vi "RW_RobotCalsALB.vi"(7 "Action":enum16{"read", "write"}(ring), 10 "Settings":T1, 11 "File Path":path=path "c:/Robot.cfg") -> (0 "error out":errorcluster, 2 "Settings out":T1)   [LabVIEW 2017]
uses:
  CtrlRefs/SettingsALB.ctl
  <vilib>/Utility/config.llb/Read Key (Double).vi
  <vilib>/Utility/config.llb/Write Key (Double).vi
  <vilib>/Utility/config.llb/NI_LVConfig.lvlib
panel:
  in  "Tab Control":enum32{"Inputs", "Outputs"}(tab)
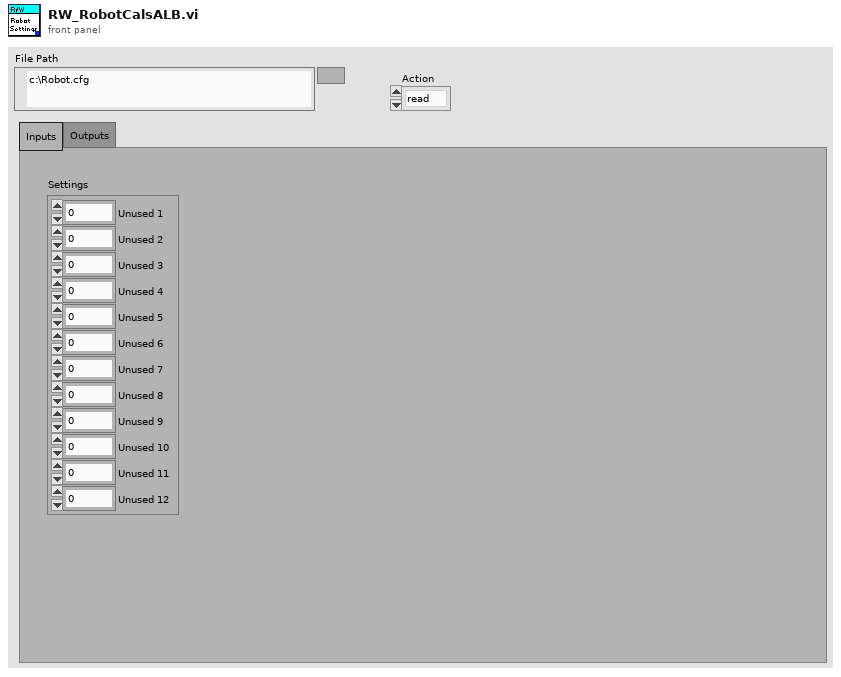
[diagram p1: front panel]
types:
  T1 = typedef "SettingsALB.ctl" = cluster{"Unused 1":dbl, "Unused 2":dbl, "Unused 3":dbl, "Unused 4":dbl, "Unused 5":dbl, "Unused 6":dbl, "Unused 7":dbl, "Unused 8":dbl, "Unused 9":dbl, "Unused 10":dbl, "Unused 11":dbl, "Unused 12":dbl}
  T2 = typedef "NI_LVConfig.lvlib/Config Data RefNum.ctl" = refnum<k1>
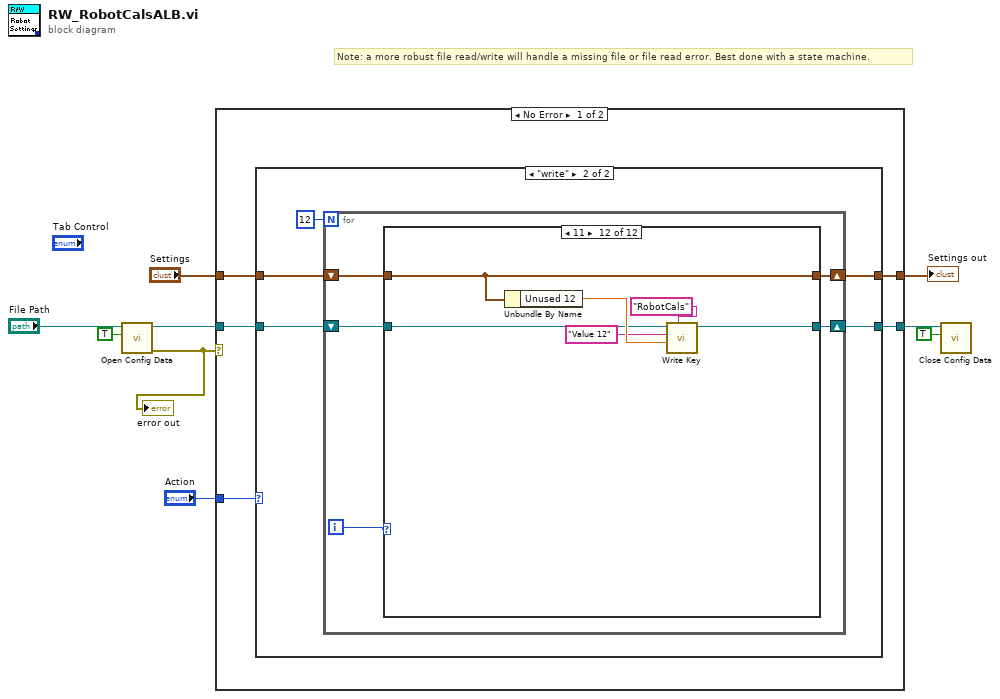
[diagram p0: block diagram]
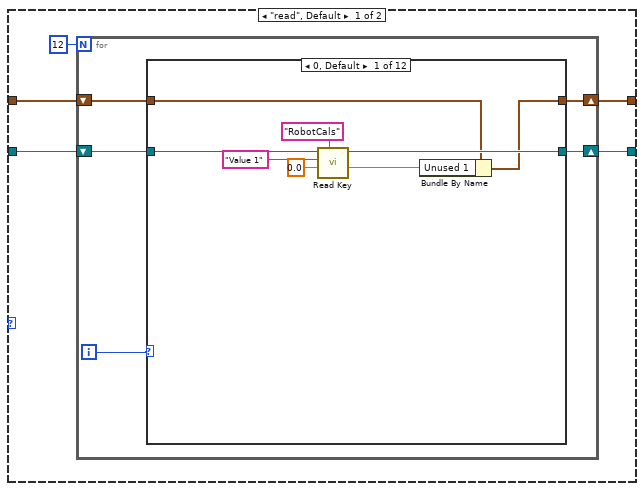
[diagram p2: hidden frame]
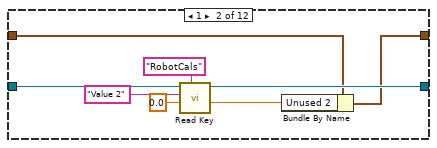
[diagram p3: hidden frame]
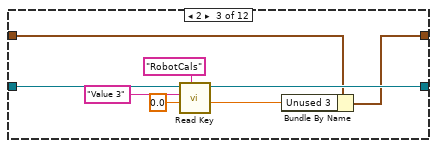
[diagram p4: hidden frame]
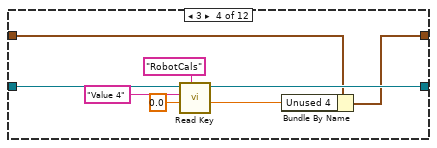
[diagram p5: hidden frame]
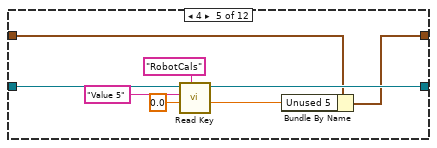
[diagram p6: hidden frame]
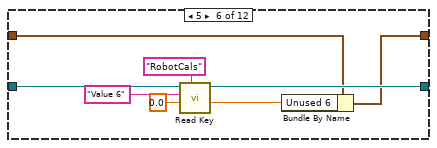
[diagram p7: hidden frame]
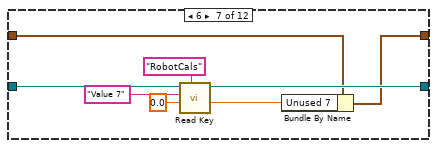
[diagram p8: hidden frame]
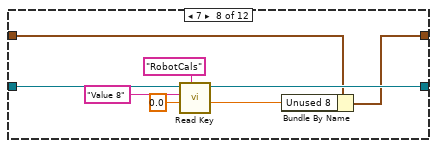
[diagram p9: hidden frame]
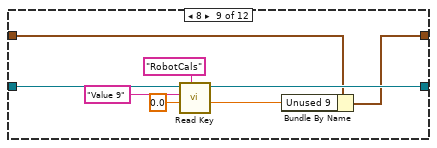
[diagram p10: hidden frame]
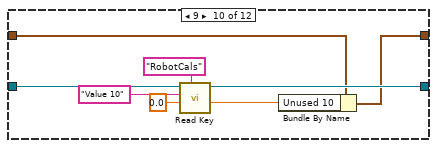
[diagram p11: hidden frame]
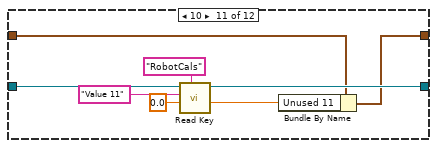
[diagram p12: hidden frame]
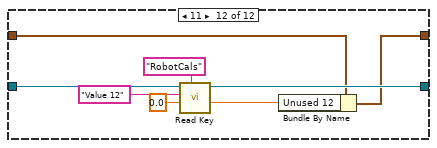
[diagram p13: hidden frame]
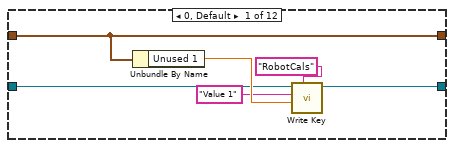
[diagram p14: hidden frame]
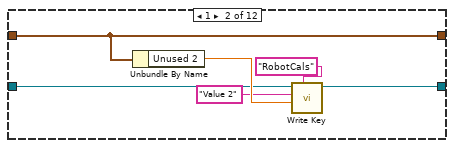
[diagram p15: hidden frame]
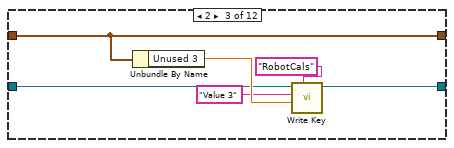
[diagram p16: hidden frame]
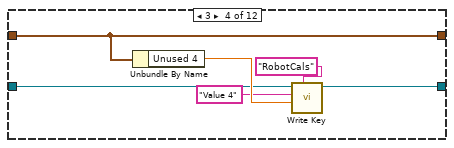
[diagram p17: hidden frame]
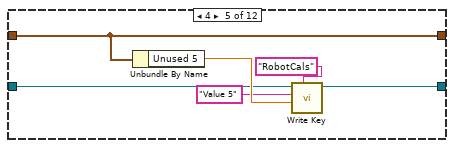
[diagram p18: hidden frame]
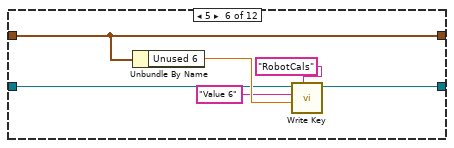
[diagram p19: hidden frame]
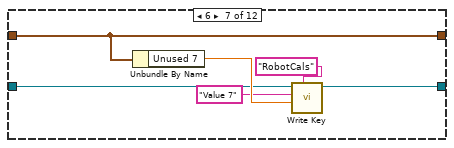
[diagram p20: hidden frame]
diagram:
  # "Note: a more robust file read/write will handle a missing file or file read error. Best done with a state machine."
  n1 = call <vilib>:"Open Config Data.vi"("create file if necessary (T)"=TRUE, "configuration file path"="File Path") -> ("error out"=w5:errorcluster, "refnum"=w7:T2)  [unwired: 7 in, 1 out]
  "error out" <- w5
  n2 = case shown="No Error" w5 {
    tunnel: "Action" -> [w14 _]
    tunnel: w7 -> [w13 w203]
    tunnel: "Settings" -> [w12 w204]
    tunnel: [w11 w204] -> w1
    tunnel: [w10 w203] -> w3
    frame No Error {
      n3 = case shown="\"write\"" w14 {
        tunnel: w13 -> [w19 w125]
        tunnel: w12 -> [w18 w124]
        tunnel: [w17 w123] -> w11
        tunnel: [w15 w121] -> w10
        frame "read", Default {
          n4 = for {
            N: 12 -> [_]
            shift-right: [w20] -> w17
            shift-left: w18 -> [w21]
            shift-right: [w22] -> w15
            shift-left: w19 -> [w23]
            i -> [w24]
            n5 = case shown="0, Default" w24 {
              tunnel: w23 -> [w28 w36 w44 w52 w60 w68 w76 w84 w92 w100 w108 w116]
              tunnel: [w27 w35 w43 w51 w59 w67 w75 w83 w91 w99 w107 w115] -> w22
              tunnel: w21 -> [w26 w34 w42 w50 w58 w66 w74 w82 w90 w98 w106 w114]
              tunnel: [w25 w33 w41 w49 w57 w65 w73 w81 w89 w97 w105 w113] -> w20
              frame 0, Default {
                n6 = call-poly <vilib>:"Read Key.vi"("section"="RobotCals", "default value"=0.0, "key"="Value 1" ("section"), "refnum"=w28) -> ("value"=w32:dbl, "refnum out"=w27:T2)  [unwired: 4 in, 2 out]
                n7 = Bundle By Name(cluster=w26, "Unused 1"=w32) -> (w25:T1)
              }
              frame 1 {
                n8 = call-poly <vilib>:"Read Key.vi"("section"="RobotCals", "default value"=0.0, "key"="Value 2" ("section"), "refnum"=w36) -> ("value"=w40:dbl, "refnum out"=w35:T2)  [unwired: 4 in, 2 out]
                n9 = Bundle By Name(cluster=w34, "Unused 2"=w40) -> (w33:T1)
              }
              frame 2 {
                n10 = call-poly <vilib>:"Read Key.vi"("section"="RobotCals", "default value"=0.0, "key"="Value 3" ("section"), "refnum"=w44) -> ("value"=w48:dbl, "refnum out"=w43:T2)  [unwired: 4 in, 2 out]
                n11 = Bundle By Name(cluster=w42, "Unused 3"=w48) -> (w41:T1)
              }
              frame 3 {
                n12 = call-poly <vilib>:"Read Key.vi"("section"="RobotCals", "default value"=0.0, "key"="Value 4" ("section"), "refnum"=w52) -> ("value"=w56:dbl, "refnum out"=w51:T2)  [unwired: 4 in, 2 out]
                n13 = Bundle By Name(cluster=w50, "Unused 4"=w56) -> (w49:T1)
              }
              frame 4 {
                n14 = call-poly <vilib>:"Read Key.vi"("section"="RobotCals", "default value"=0.0, "key"="Value 5" ("section"), "refnum"=w60) -> ("value"=w64:dbl, "refnum out"=w59:T2)  [unwired: 4 in, 2 out]
                n15 = Bundle By Name(cluster=w58, "Unused 5"=w64) -> (w57:T1)
              }
              frame 5 {
                n16 = call-poly <vilib>:"Read Key.vi"("section"="RobotCals", "default value"=0.0, "key"="Value 6" ("section"), "refnum"=w68) -> ("value"=w72:dbl, "refnum out"=w67:T2)  [unwired: 4 in, 2 out]
                n17 = Bundle By Name(cluster=w66, "Unused 6"=w72) -> (w65:T1)
              }
              frame 6 {
                n18 = call-poly <vilib>:"Read Key.vi"("section"="RobotCals", "default value"=0.0, "key"="Value 7" ("section"), "refnum"=w76) -> ("value"=w80:dbl, "refnum out"=w75:T2)  [unwired: 4 in, 2 out]
                n19 = Bundle By Name(cluster=w74, "Unused 7"=w80) -> (w73:T1)
              }
              frame 7 {
                n20 = call-poly <vilib>:"Read Key.vi"("section"="RobotCals", "default value"=0.0, "key"="Value 8" ("section"), "refnum"=w84) -> ("value"=w88:dbl, "refnum out"=w83:T2)  [unwired: 4 in, 2 out]
                n21 = Bundle By Name(cluster=w82, "Unused 8"=w88) -> (w81:T1)
              }
              frame 8 {
                n22 = call-poly <vilib>:"Read Key.vi"("section"="RobotCals", "default value"=0.0, "key"="Value 9" ("section"), "refnum"=w92) -> ("value"=w96:dbl, "refnum out"=w91:T2)  [unwired: 4 in, 2 out]
                n23 = Bundle By Name(cluster=w90, "Unused 9"=w96) -> (w89:T1)
              }
              frame 9 {
                n24 = call-poly <vilib>:"Read Key.vi"("section"="RobotCals", "default value"=0.0, "key"="Value 10" ("section"), "refnum"=w100) -> ("value"=w104:dbl, "refnum out"=w99:T2)  [unwired: 4 in, 2 out]
                n25 = Bundle By Name(cluster=w98, "Unused 10"=w104) -> (w97:T1)
              }
              frame 10 {
                n26 = call-poly <vilib>:"Read Key.vi"("section"="RobotCals", "default value"=0.0, "key"="Value 11" ("section"), "refnum"=w108) -> ("value"=w112:dbl, "refnum out"=w107:T2)  [unwired: 4 in, 2 out]
                n27 = Bundle By Name(cluster=w106, "Unused 11"=w112) -> (w105:T1)
              }
              frame 11 {
                n28 = call-poly <vilib>:"Read Key.vi"("section"="RobotCals", "default value"=0.0, "key"="Value 12" ("section"), "refnum"=w116) -> ("value"=w120:dbl, "refnum out"=w115:T2)  [unwired: 4 in, 2 out]
                n29 = Bundle By Name(cluster=w114, "Unused 12"=w120) -> (w113:T1)
              }
            }
          }
        }
        frame "write" {
          n30 = for {
            N: 12 -> [_]
            shift-right: [w128] -> w123
            shift-left: w124 -> [w129]
            shift-right: [w126] -> w121
            shift-left: w125 -> [w127]
            i -> [w130]
            n31 = case shown="11" w130 {
              tunnel: w129 -> [w133 w139 w145 w151 w157 w163 w169 w175 w181 w187 w193 w199]
              tunnel: [w133 w139 w145 w151 w157 w163 w169 w175 w181 w187 w193 w199] -> w128
              tunnel: w127 -> [w132 w138 w144 w150 w156 w162 w168 w174 w180 w186 w192 w198]
              tunnel: [w131 w137 w143 w149 w155 w161 w167 w173 w179 w185 w191 w197] -> w126
              frame 0, Default {
                n32 = Unbundle By Name(w133) -> ("Unused 1"=w136:dbl)
                n33 = call-poly <vilib>:"Write Key.vi"("section"="RobotCals", "value"=w136, "key"="Value 1" ("section"), "refnum"=w132) -> ("refnum out"=w131:T2)  [unwired: 5 in, 2 out]
              }
              frame 1 {
                n34 = Unbundle By Name(w139) -> ("Unused 2"=w142:dbl)
                n35 = call-poly <vilib>:"Write Key.vi"("section"="RobotCals", "value"=w142, "key"="Value 2" ("section"), "refnum"=w138) -> ("refnum out"=w137:T2)  [unwired: 5 in, 2 out]
              }
              frame 2 {
                n36 = Unbundle By Name(w145) -> ("Unused 3"=w148:dbl)
                n37 = call-poly <vilib>:"Write Key.vi"("section"="RobotCals", "value"=w148, "key"="Value 3" ("section"), "refnum"=w144) -> ("refnum out"=w143:T2)  [unwired: 5 in, 2 out]
              }
              frame 3 {
                n38 = Unbundle By Name(w151) -> ("Unused 4"=w154:dbl)
                n39 = call-poly <vilib>:"Write Key.vi"("section"="RobotCals", "value"=w154, "key"="Value 4" ("section"), "refnum"=w150) -> ("refnum out"=w149:T2)  [unwired: 5 in, 2 out]
              }
              frame 4 {
                n40 = Unbundle By Name(w157) -> ("Unused 5"=w160:dbl)
                n41 = call-poly <vilib>:"Write Key.vi"("section"="RobotCals", "value"=w160, "key"="Value 5" ("section"), "refnum"=w156) -> ("refnum out"=w155:T2)  [unwired: 5 in, 2 out]
              }
              frame 5 {
                n42 = Unbundle By Name(w163) -> ("Unused 6"=w166:dbl)
                n43 = call-poly <vilib>:"Write Key.vi"("section"="RobotCals", "value"=w166, "key"="Value 6" ("section"), "refnum"=w162) -> ("refnum out"=w161:T2)  [unwired: 5 in, 2 out]
              }
              frame 6 {
                n44 = Unbundle By Name(w169) -> ("Unused 7"=w172:dbl)
                n45 = call-poly <vilib>:"Write Key.vi"("section"="RobotCals", "value"=w172, "key"="Value 7" ("section"), "refnum"=w168) -> ("refnum out"=w167:T2)  [unwired: 5 in, 2 out]
              }
              frame 7 {
                n46 = Unbundle By Name(w175) -> ("Unused 8"=w178:dbl)
                n47 = call-poly <vilib>:"Write Key.vi"("section"="RobotCals", "value"=w178, "key"="Value 8" ("section"), "refnum"=w174) -> ("refnum out"=w173:T2)  [unwired: 5 in, 2 out]
              }
              frame 8 {
                n48 = Unbundle By Name(w181) -> ("Unused 9"=w184:dbl)
                n49 = call-poly <vilib>:"Write Key.vi"("section"="RobotCals", "value"=w184, "key"="Value 9" ("section"), "refnum"=w180) -> ("refnum out"=w179:T2)  [unwired: 5 in, 2 out]
              }
              frame 9 {
                n50 = Unbundle By Name(w187) -> ("Unused 10"=w190:dbl)
                n51 = call-poly <vilib>:"Write Key.vi"("section"="RobotCals", "value"=w190, "key"="Value 10" ("section"), "refnum"=w186) -> ("refnum out"=w185:T2)  [unwired: 5 in, 2 out]
              }
              frame 10 {
                n52 = Unbundle By Name(w193) -> ("Unused 11"=w196:dbl)
                n53 = call-poly <vilib>:"Write Key.vi"("section"="RobotCals", "value"=w196, "key"="Value 11" ("section"), "refnum"=w192) -> ("refnum out"=w191:T2)  [unwired: 5 in, 2 out]
              }
              frame 11 {
                n54 = Unbundle By Name(w199) -> ("Unused 12"=w202:dbl)
                n55 = call-poly <vilib>:"Write Key.vi"("section"="RobotCals", "value"=w202, "key"="Value 12" ("section"), "refnum"=w198) -> ("refnum out"=w197:T2)  [unwired: 5 in, 2 out]
              }
            }
          }
        }
      }
    }
    frame Error {
    }
  }
  "Settings out" <- w1
  n56 = call <vilib>:"Close Config Data.vi"("write file if changed (T)"=TRUE, "refnum"=w3) -> ()  [unwired: 8 in, 2 out]
